vi "DAQmx Create Channel (CI-Duty Cycle).vi"(0 "task in":refnum<k21>, 1 "maximum frequency":dbl=10000.0 format="%0.6f", 2 "minimum frequency":dbl=2.0 format="%0.6f", 5 "counter":tag, 7 "name to assign":string, 11 "error in":errorcluster, 12 "custom scale name":tag, 13 "starting edge":i32(ring)=10280 items=["Rising"=10280, "Falling"=10171]) -> (4 "task out":refnum<k21>, 15 "error out":errorcluster)   [LabVIEW 2020]
doc: "Creates channel(s) to duty cycle of a digital pulse. Connect the input signal to the default input terminal of the counter unless you select a different input terminal. With the exception of devices that support multi-counter tasks, you can create only one counter input channel at a time with this VI because a task can contain only one counter input channel. To read from multiple counters simultaneously, use a separate task for each counter."
uses:
  nilvaiu.dll
panel:
  # "input limits"
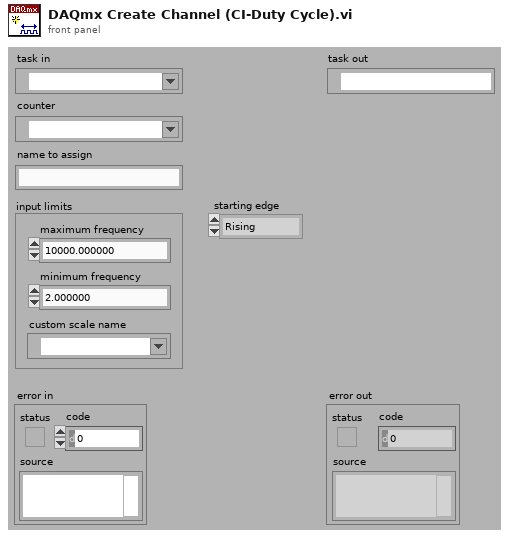
[diagram p1: front panel]
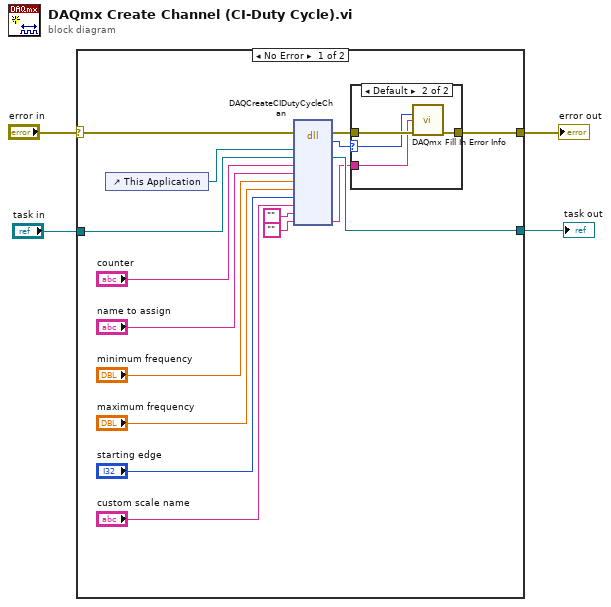
[diagram p0: block diagram]
diagram:
  n1 = case shown="No Error" "error in" {
    selector: "error in" -> [w6 w27]
    tunnel: "task in" -> [w20 w26]
    tunnel: [w19 w26] -> w3
    tunnel: [w18 w27] -> w2
    frame No Error {
      n2 = control-ref of="This Application"() -> (w14:refnum<vi>)
      n3 = dll-call lib="nilvaiu.*" fn="DAQCreateCIDutyCycleChan"(error in=w6, "lvAppRef"=w14, "refObjPtr"=w20, "counter"="counter", "channelNameIn"="name to assign", "minFreq"="minimum frequency", "maxFreq"="maximum frequency", "startingEdge"="starting edge", "customScaleName"="custom scale name", "channelNamesOut"="", "extendedErrorInfo"="") -> (error out=w17:errorcluster, "return type"=w16:i32, "refObjPtr"=w19:refnum<k21>, "extendedErrorInfo"=w15:string)  [unwired: 10 in, 1 out]
      n4 = case shown="Default" w16 {
        selector: w16 -> [_ w23]
        tunnel: w17 -> [w21 w25]
        tunnel: [w21 w24] -> w18
        tunnel: w15 -> [_ w22]
        frame 0 {
        }
        frame Default {
          n5 = call "DAQmx Fill In Error Info.vi"("status code"=w23, "extended error info"=w22, "error in"=w25) -> ("error out"=w24:errorcluster)  [unwired: 1 in, 11 out]
        }
      }
    }
    frame Error {
    }
  }
  "error out" <- w2
  "task out" <- w3
